vi "Config Data Get File Path.vi"(8 "error in (no error)":errorcluster caption="Fehler (Eingang, kein Fehler)", 11 "config data reference":T1 caption="Konfigurationsdaten-Referenz") -> (0 "error out":errorcluster caption="Fehler (Ausgang)", 2 "file path":path caption="Dateipfad", 3 "config data reference out":T1 caption="Konfigurationsdaten-Referenz (Ausgang)")   [LabVIEW 2009]
doc: "Holt die Dateipfad-Eigenschaft eines Konfigurationsdaten-Objekts."
uses:
  <vilib>/Utility/config.llb/Config Data RefNum.ctl
  Config Data Registry Functions.ctl
  <vilib>/Utility/config.llb/NI_LVConfig.lvlib
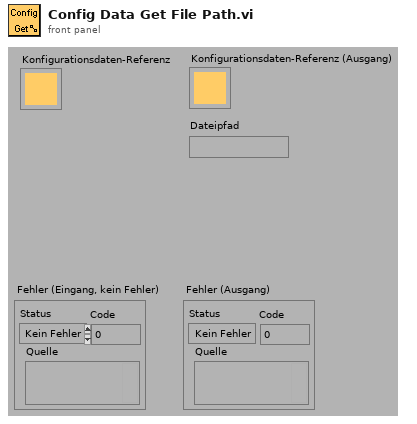
[diagram p1: front panel]
types:
  T1 = typedef "NI_LVConfig.lvlib/Config Data RefNum.ctl" = refnum<k1>
  T2 = typedef "Config Data Registry Functions.ctl" = enum16{"reset", "register", "get data", "get section", "set data", "unregister", "test", "get objects"}
  T3 = typedef "Config Data.ctl" = cluster{"file path":path, "data":T4[], "section names":string[]}
  T4 = typedef "Config Data Section.ctl" = cluster{"keys":string[], "values":string[]}
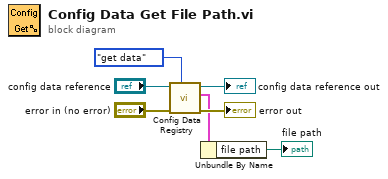
[diagram p0: block diagram]
diagram:
  n1 = call "Config Data Registry.vi"("function (get data)"=Config_Data_Registry_Functions."get data", "error in (no error)"="error in (no error)", "config data"="config data reference") -> ("error out"=→"error out":errorcluster, 2:"config data out"=w3:T3, 3:"config data out"=→"config data reference out":T1)  [unwired: 2 in, 4 out]
  n2 = Unbundle By Name(w3) -> ("file path"=→"file path":path)
